vi "Controller Operation Mode.vi"() -> ()   [LabVIEW 2011, in "Controller Global Variables.lvlib"]
uses:
  Controller Global Variables.lvlib
panel:
  in  "Controller Operation Mode":T1(ring)=enum."Manual Mode"
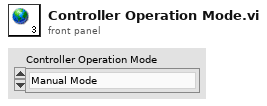
[diagram p1: front panel]
types:
  T1 = enum16{"Idle Mode", "Error Mode", "Manual Mode", "FOFB Mode", "RMM Mode"}
diagram:
